vi "Repeatability Math.vi"(0 "Calibration Points in":T1[](array[typedef]), 11 "error in (no error)":errorcluster) -> (4 "Calibration Points out":T1[](array[typedef]), 6 "Current Calibration Point":T1, 8 "Next Calibration Point":T1, 10 "Numeric":dbl, 15 "error out":errorcluster)   [LabVIEW 2026, in "Analysis.lvlib"]
uses:
  Analysis.lvlib
  controls/Messaging Payloads/Calibration Point Table Insert.ctl
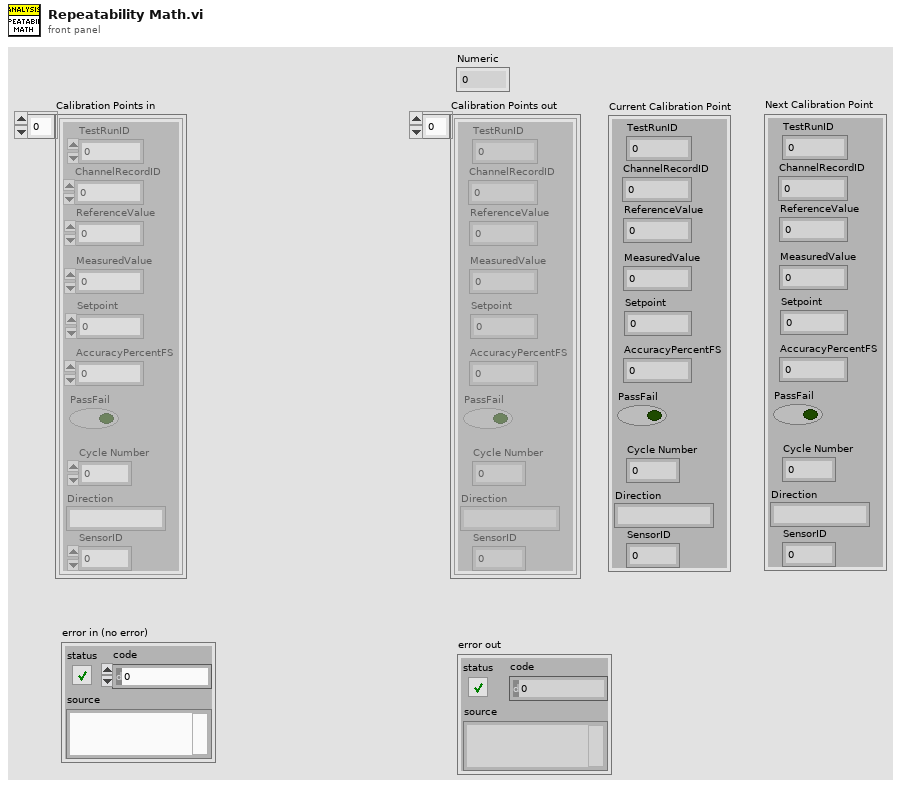
[diagram p1: front panel]
types:
  T1 = typedef "Calibration Point Table Insert.ctl" = cluster{"TestRunID":i32, "ChannelRecordID":i32, "Setpoint":dbl, "MeasuredValue":dbl, "AccuracyPercentFS":dbl, "PassFail":bool, "ReferenceValue":dbl, "Cycle Number":i32, "Direction":string, "SensorID":i32}
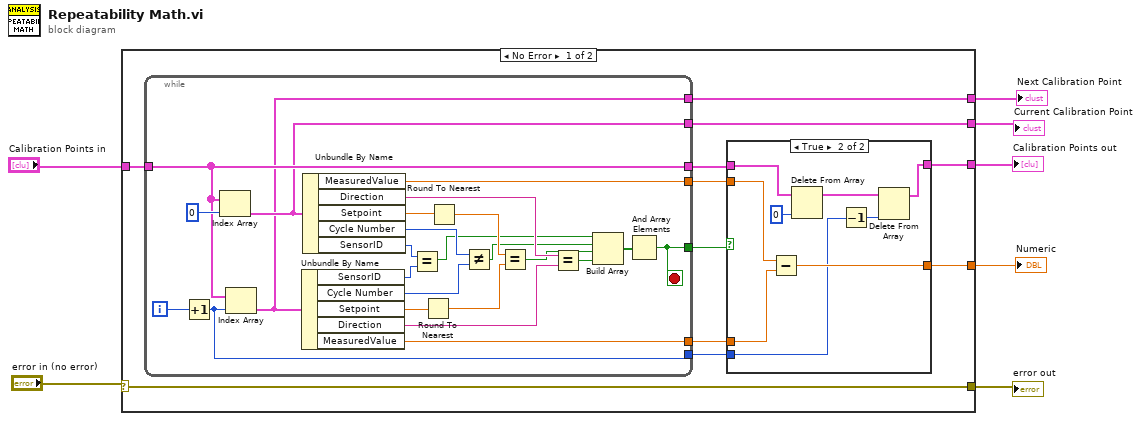
[diagram p0: block diagram]
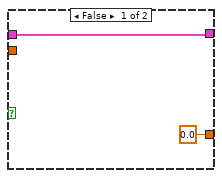
[diagram p2: hidden frame]
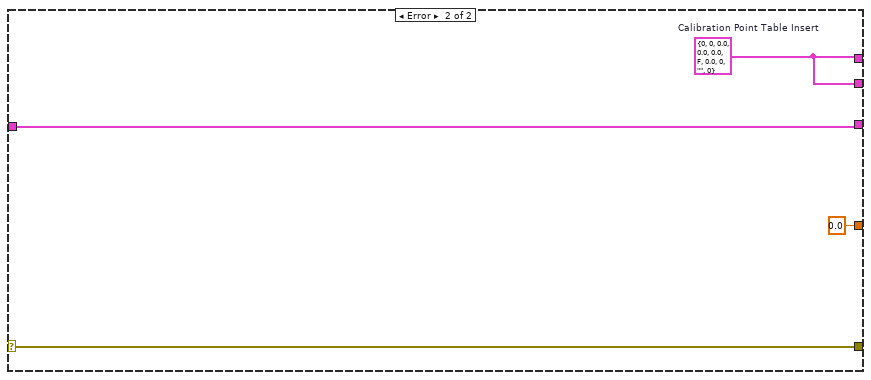
[diagram p3: hidden frame]
diagram:
  n1 = case shown="No Error" "error in (no error)" {
    selector: "error in (no error)" -> [w8 w55]
    tunnel: [w17 w56] -> w7
    tunnel: [w16 w56] -> w6
    tunnel: [w15 0.0] -> w5
    tunnel: [w14 w57] -> w4
    tunnel: "Calibration Points in" -> [w9 w57]
    tunnel: [w8 w55] -> w1
    frame No Error {
      n2 = while {
        tunnel: w9 -> [w34]
        tunnel: [w35] -> w18
        tunnel: [w37] -> w10
        tunnel: [w36] -> w11
        tunnel: [w34] -> w13
        tunnel: [w32] -> w12
        tunnel: [w31] -> w16
        tunnel: [w30] -> w17
        i -> [w33]
        stop <- w35 stop-if-true
        n3 = Increment(x=w33) -> (x+1=w32:i32)
        n4 = Index Array(array=w34, index=0) -> (element=w31:T1)
        n5 = Index Array(array=w34, index=w32) -> (element=w30:T1)
        n6 = Unbundle By Name(w30) -> ("SensorID"=w51:i32, "Cycle Number"=w49:i32, "Setpoint"=w46:dbl, "Direction"=w43:string, "MeasuredValue"=w36:dbl)
        n7 = Unbundle By Name(w31) -> ("MeasuredValue"=w37:dbl, "Direction"=w44:string, "Setpoint"=w48:dbl, "Cycle Number"=w50:i32, "SensorID"=w52:i32)
        n8 = Equal?(x=w52, y=w51) -> (x = y?=w39:bool)
        n9 = Round To Nearest(number=w46) -> (nearest integer value=w45:dbl)
        n10 = Round To Nearest(number=w48) -> (nearest integer value=w47:dbl)
        n11 = Not Equal?(x=w50, y=w49) -> (x != y?=w40:bool)
        n12 = Equal?(x=w47, y=w45) -> (x = y?=w41:bool)
        n13 = Equal?(x=w44, y=w43) -> (x = y?=w42:bool)
        n14 = Build Array(w39, w40, w41, w42) -> (w38:bool[])
        n15 = And Array Elements(Boolean array=w38) -> (logical AND=w35:bool)
      }
      n16 = case shown="True" w18 {
        tunnel: [w20 w23] -> w14
        tunnel: w13 -> [w20 w29]
        tunnel: w10 -> [_ w26]
        tunnel: w11 -> [_ w27]
        tunnel: [0.0 w25] -> w15
        tunnel: w12 -> [_ w22]
        frame False {
        }
        frame True {
          n17 = Subtract(x=w26, y=w27) -> (x-y=w25:dbl)
          n18 = Delete From Array(array=w29, index=0) -> (array with subset deleted=w24:T1[])  [unwired: 1 in, 1 out]
          n19 = Decrement(x=w22) -> (x-1=w21:i32)
          n20 = Delete From Array(array=w24, index=w21) -> (array with subset deleted=w23:T1[])  [unwired: 1 in, 1 out]
        }
      }
    }
    frame Error {
      w56 = T1 {"TestRunID"=0, "ChannelRecordID"=0, "Setpoint"=0.0, "MeasuredValue"=0.0, "AccuracyPercentFS"=0.0, "PassFail"=FALSE, "ReferenceValue"=0.0, "Cycle Number"=0, "Direction"="", "SensorID"=0}  # Calibration Point Table Insert
    }
  }
  "Next Calibration Point" <- w7
  "Current Calibration Point" <- w6
  "Numeric" <- w5
  "Calibration Points out" <- w4
  "error out" <- w1
